vi "PM5000_PowerQualityLogData.vi"(8 "error in":errorcluster, 11 "Network Path":string="172.22.26.202") -> (0 "error out":errorcluster, 1 "PQ_Log array out":sgl[](array[numeric]), 2 "PowerQualityLog out":T1, 3 "Network Path out":string="192.168.169.1")   [LabVIEW 2018]
doc: "Lee la tabla de memoria RealTime_VIF_Power del equipo PowerMonitor 5000, ademas filtra y ordena las variables de interez de la tabla de memoria.\n\nLee las siguientes variables de la tabla RealTime_VIF_Power:\n\n*V1_V2_Volts\n*V2_V3_Volts\n*V3_V1_Volts\n*I1_Amps\n*I2_Amps\n*I3_Amps\n*Frequency_Hz\n*Total_kW\n*Total_kVAR\n*Total_kVA\n*Total_True_PF\n*Total_Disp_PF"
uses:
  <vilib>/ethernetip/ethernetip.llb/EthernetIP SLC500 Read Float.vi
  <vilib>/ethernetip/ethernetip.lvlib
panel:
  out "Record_Identifier":sgl
  out "SubEVento":string
  out "Evento":string
  out "Local_Timestamp_Sec_mS":sgl
  out "Local_Timestamp_Hr_Min":sgl
  out "Local_Timestamp_Mth_Day":sgl
  out "Local_Timestamp_Year":sgl
  out "Sub_Event_Code":sgl
  out "Event_Type":sgl
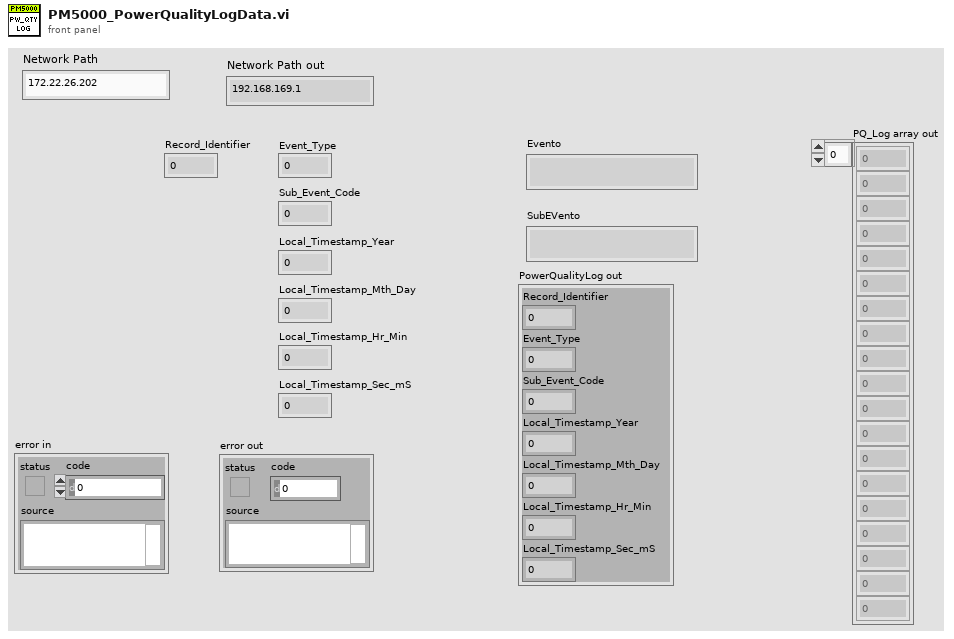
[diagram p1: front panel]
types:
  T1 = cluster{"Record_Identifier":sgl, "Event_Type":sgl, "Sub_Event_Code":sgl, "Local_Timestamp_Year":sgl, "Local_Timestamp_Mth_Day":sgl, "Local_Timestamp_Hr_Min":sgl, "Local_Timestamp_Sec_mS":sgl}
  T2 = cluster{"Real Power (kW)":cluster{"L1_kW":sgl, "L2_kW":sgl, "L3_kW":sgl, "Total_kW":sgl}, "Reactive Power (kVAR)":cluster{"L1_kVAR":sgl, "L2_kVAR":sgl, "L3_kVAR":sgl, "Total_kVAR":sgl}, "Aparent Power (kVA)":cluster{"L1_kVA":sgl, "L2_kVA":sgl, "L3_kVA":sgl, "Total_kVA":sgl}, "Power Factor (%)":cluster{"L1_PF":sgl, "L2_PF":sgl, "L3_PF":sgl, "Total_PF":sgl}}
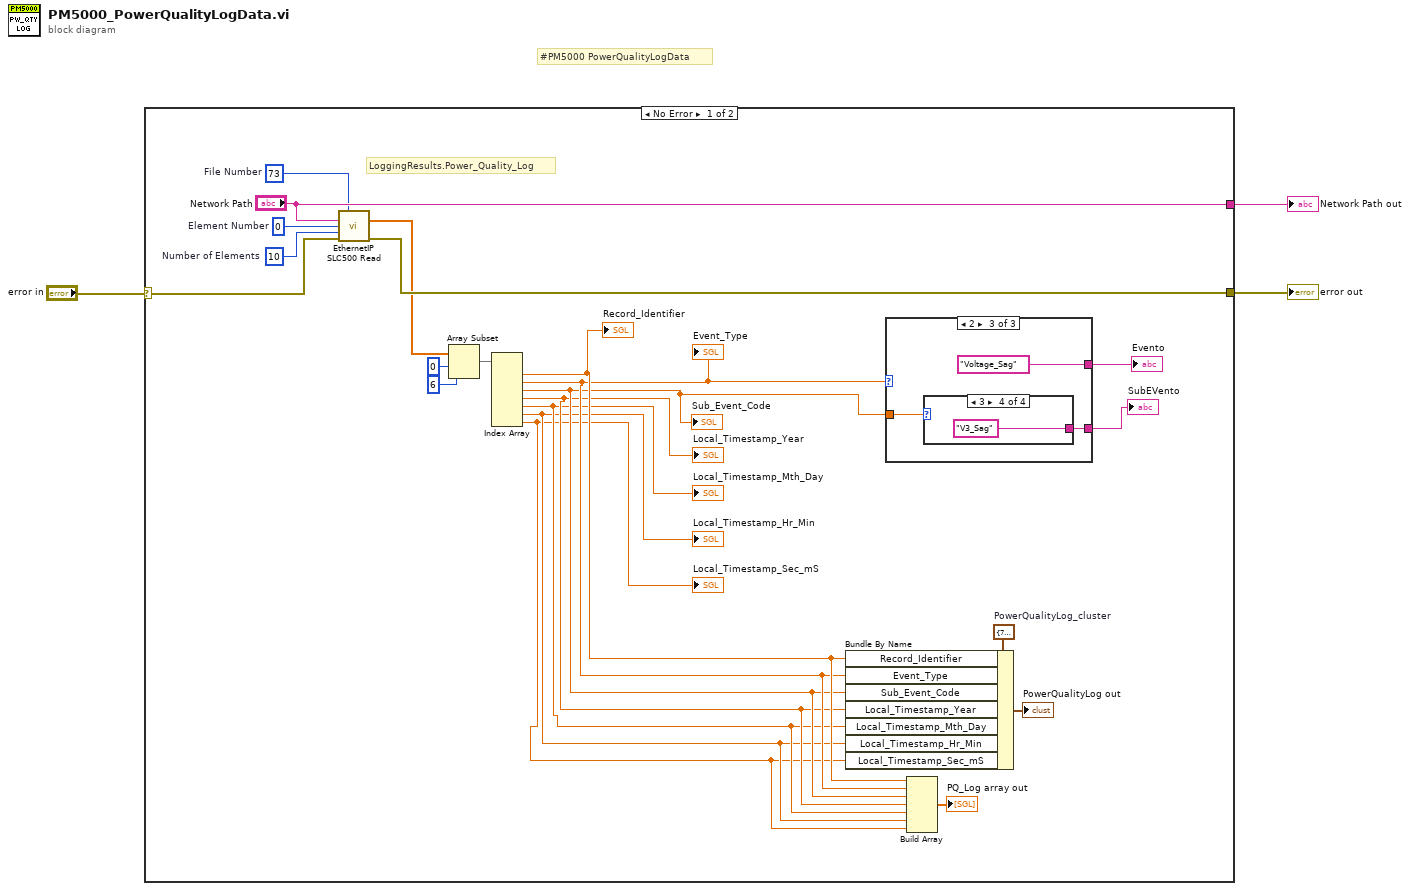
[diagram p0: block diagram]
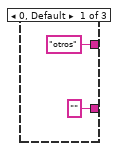
[diagram p2: hidden frame]
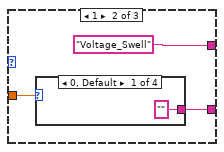
[diagram p3: hidden frame]
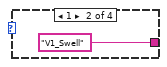
[diagram p4: hidden frame]
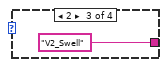
[diagram p5: hidden frame]
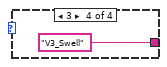
[diagram p6: hidden frame]
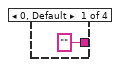
[diagram p7: hidden frame]
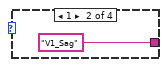
[diagram p8: hidden frame]
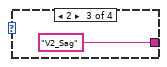
[diagram p9: hidden frame]
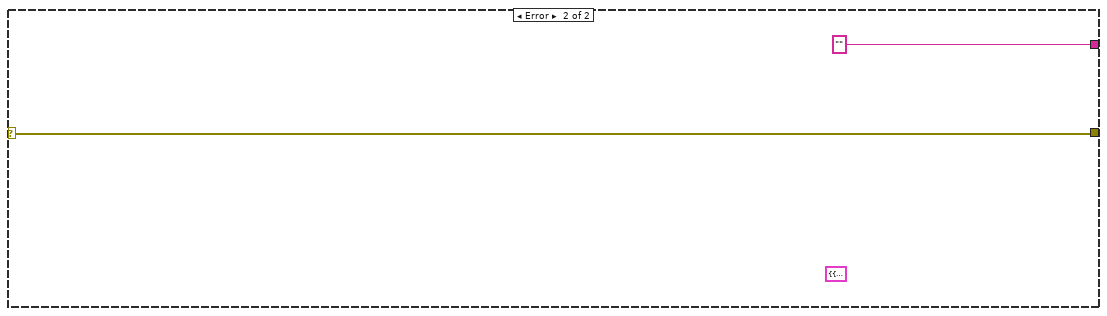
[diagram p10: hidden frame]
diagram:
  # "#PM5000 PowerQualityLogData"
  n1 = case shown="No Error" "error in" {
    selector: "error in" -> [w19 w42]
    tunnel: [w25 w42] -> w3
    tunnel: ["Network Path" "" ("Network Path")] -> w2
    frame No Error {
      w13 = T1 {"Record_Identifier"=74.0, "Event_Type"=13.0, "Sub_Event_Code"=1.0, "Local_Timestamp_Year"=2019.0, "Local_Timestamp_Mth_Day"=128.0, "Local_Timestamp_Hr_Min"=1446.0, "Local_Timestamp_Sec_mS"=15503.0}  # PowerQualityLog_cluster
      w21 = u32 10  # Number of Elements
      w23 = u16 73  # File Number
      w22 = u16 0  # Element Number
      # "LoggingResults.Power_Quality_Log"
      n2 = call-poly <vilib>:"EthernetIP SLC500 Read.vi"("File Number"=w23, "Network Path"="Network Path", "Element Number"=w22, "Number of Elements"=w21, "error in"=w19) -> ("Data"=w15:sgl[], "error out"=w25:errorcluster)  [unwired: 8 in, 1 out]
      n3 = Array Subset(array=w15, index=0, length=6) -> (w14:sgl[])
      n4 = Index Array(array=w14) -> (element #1=w11:sgl, element #2=w10:sgl, element #3=w9:sgl, element #4=w8:sgl, element #5=w7:sgl, element #6=w6:sgl, element #7=w5:sgl)  [unwired: 7 in]
      "Event_Type" <- w10
      "Sub_Event_Code" <- w9
      "Local_Timestamp_Year" <- w8
      "Local_Timestamp_Mth_Day" <- w7
      "Local_Timestamp_Hr_Min" <- w6
      "Local_Timestamp_Sec_mS" <- w5
      "Record_Identifier" <- w11
      n5 = Bundle By Name(cluster=w13, "Record_Identifier"=w11, "Event_Type"=w10, "Sub_Event_Code"=w9, "Local_Timestamp_Year"=w8, "Local_Timestamp_Mth_Day"=w7, "Local_Timestamp_Hr_Min"=w6, "Local_Timestamp_Sec_mS"=w5) -> (→"PowerQualityLog out":T1)
      n6 = case shown="2" w10 {
        tunnel: ["otros" "Voltage_Swell" "Voltage_Sag"] -> w17
        tunnel: w9 -> [_ w28 w36]
        tunnel: ["" w29 w35] -> w16
        frame 0, Default {
        }
        frame 1 {
          n7 = case shown="0, Default" w28 {
            tunnel: ["" "V1_Swell" "V2_Swell" "V3_Swell"] -> w29
            frame 0, Default {
            }
            frame 1 {
            }
            frame 2 {
            }
            frame 3 {
            }
          }
        }
        frame 2 {
          n8 = case shown="3" w36 {
            tunnel: ["" "V1_Sag" "V2_Sag" "V3_Sag"] -> w35
            frame 0, Default {
            }
            frame 1 {
            }
            frame 2 {
            }
            frame 3 {
            }
          }
        }
      }
      "Evento" <- w17
      "SubEVento" <- w16
      n9 = Build Array(w11, w10, w9, w8, w7, w6, w5) -> (→"PQ_Log array out":sgl[])
    }
    frame Error {
      (unwired) T2 {"Real Power (kW)"={"L1_kW"=0.0, "L2_kW"=0.0, "L3_kW"=0.0, "Total_kW"=0.0}, "Reactive Power (kVAR)"={"L1_kVAR"=0.0, "L2_kVAR"=0.0, "L3_kVAR"=0.0, "Total_kVAR"=0.0}, "Aparent Power (kVA)"={"L1_kVA"=0.0, "L2_kVA"=0.0, "L3_kVA"=0.0, "Total_kVA"=0.0}, "Power Factor (%)"={"L1_PF"=0.0, "L2_PF"=0.0, "L3_PF"=0.0, "Total_PF"=0.0}} ("Power Meter")
    }
  }
  "error out" <- w3
  "Network Path out" <- w2
